vi "Ejercicio_1_2.vi"() -> ()   [LabVIEW 2020]
panel:
  in  "Botón de parada":bool
  out "LED":bool
  in  "Boton":bool
  out "Indicador":dbl(knob) scale=0.0..30.0
  in  "Perilla":dbl(knob) scale=0.0..30.0
  out "Edad mostrada":i32(slide) scale=0.0..80.0
  in  "Edad":i32
  out "String indicador":string
  in  "String control":string
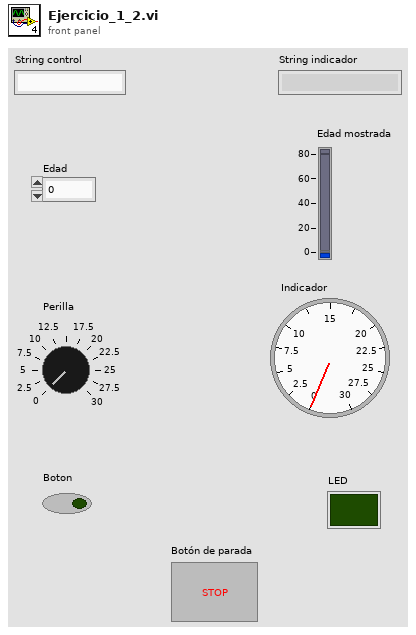
[diagram p1: front panel]
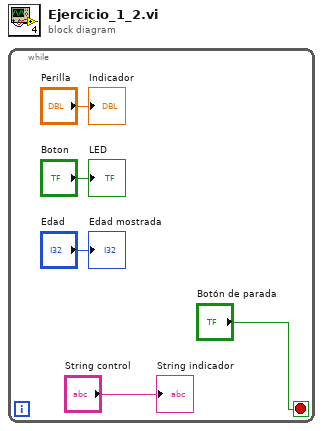
[diagram p0: block diagram]
diagram:
  n1 = while {
    stop <- "Botón de parada" stop-if-true
    "String indicador" <- "String control"
    "Edad mostrada" <- "Edad"
    "Indicador" <- "Perilla"
    "LED" <- "Boton"
  }
